vi "test3.vi"() -> ()   [LabVIEW 2013]
uses:
  LightField Automation.lvclass
panel:
  out "LightField Automation out":refnum<class "LightField Automation.lvclass">
  in  "Gate Mode":string(combo)
  in  "Intensifier Gain":i32=1
  in  "ExperimentName":string="Experiment2"
  in  "?":bool
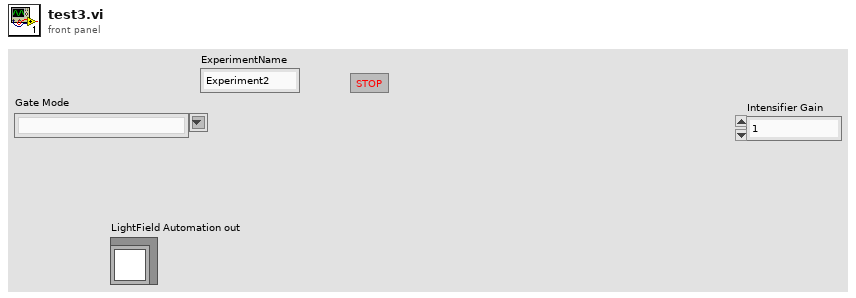
[diagram p1: front panel]
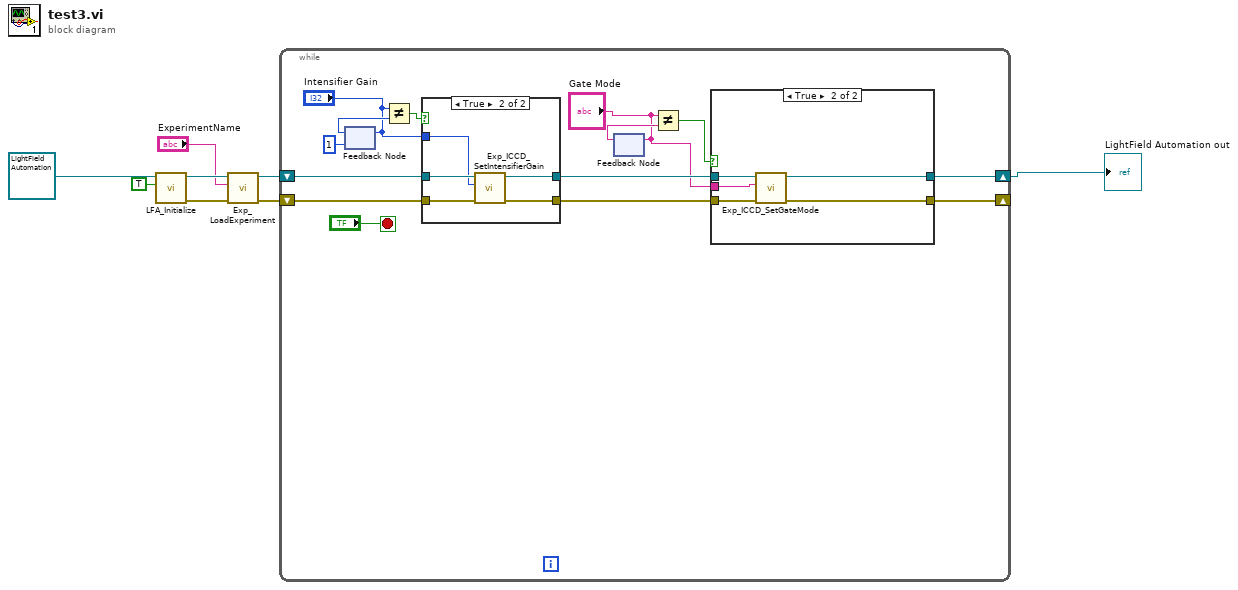
[diagram p0: block diagram]
diagram:
  n1 = call "LFA_Initialize.vi"("Is Visible?"=TRUE, "LightField Automation in"=refnum<class "LightField Automation.lvclass"> refnum ("LightField Automation.lvclass")) -> ("error out"=w5:errorcluster, "LightField Automation out"=w6:refnum<class "LightField Automation.lvclass">)  [unwired: 8 in]
  n2 = call "Exp_LoadExperiment.vi"("error in (no error)"=w5, "ExperimentName"="ExperimentName", "LightField Automation in"=w6) -> ("error out"=w4:errorcluster, "LightField Automation out"=w3:refnum<class "LightField Automation.lvclass">)  [unwired: 7 in]
  n3 = while {
    shift-right: [w13] -> w1
    shift-left: w3 -> [w19]
    shift-right: [w12] -> _
    shift-left: w4 -> [w18]
    stop <- "?" stop-if-true
    n4 = feedback #1(1 ("Intensifier Gain")) -> (w21:i32)
    n5 = feedback-in #1("Intensifier Gain") -> ()
    n6 = Not Equal?(x="Intensifier Gain", y=w21) -> (x != y?=w20:bool)
    n7 = case shown="True" w20 {
      tunnel: "Intensifier Gain" -> [_ w32]
      tunnel: w19 -> [w30 w36]
      tunnel: w18 -> [w31 w35]
      tunnel: [w30 w33] -> w15
      tunnel: [w31 w34] -> w14
      frame False {
      }
      frame True {
        n8 = call "Exp_ICCD_SetIntensifierGain.vi"("error in (no error)"=w35, "Intensifier Gain"=w32, "LightField Automation in"=w36) -> ("error out"=w34:errorcluster, "LightField Automation out"=w33:refnum<class "LightField Automation.lvclass">)  [unwired: 7 in]
      }
    }
    n9 = feedback #2() -> (w11:string)  [unwired: 1 in]
    n10 = feedback-in #2("Gate Mode") -> ()
    n11 = Not Equal?(x="Gate Mode", y=w11) -> (x != y?=w10:bool)
    n12 = case shown="True" w10 {
      tunnel: w15 -> [w23 w29]
      tunnel: w14 -> [w24 w28]
      tunnel: [w23 w26] -> w13
      tunnel: [w24 w25] -> w12
      tunnel: "Gate Mode" -> [_ w27]
      frame False {
      }
      frame True {
        n13 = call "Exp_ICCD_SetGateMode.vi"("error in (no error)"=w28, "Gate Mode"=w27, "LightField Automation in"=w29) -> ("error out"=w25:errorcluster, "LightField Automation out"=w26:refnum<class "LightField Automation.lvclass">)  [unwired: 7 in]
      }
    }
  }
  "LightField Automation out" <- w1
